vi "TDMS logging.vi"(8 "error in (no error)":errorcluster, 9 "Data":ext[][](array[numeric]), 10 "Default TDMS path":string, 11 "logg ON/OFF":bool) -> (0 "error out":errorcluster, 3 "Logg path":path)   [LabVIEW 2014]
uses:
  Ctrls/TDMS logg state.ctl
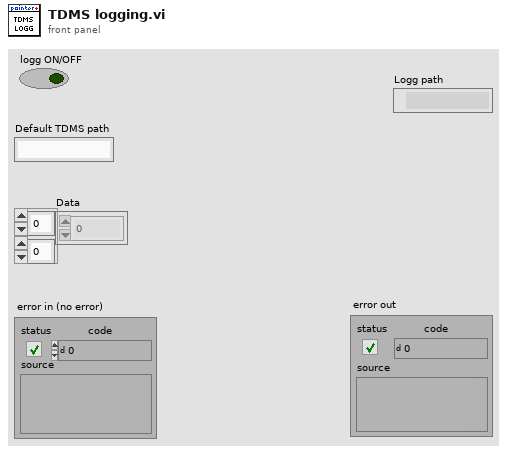
[diagram p1: front panel]
types:
  T1 = typedef "TDMS logg state.ctl" = enum16{"start", "logg", "end", "none"}
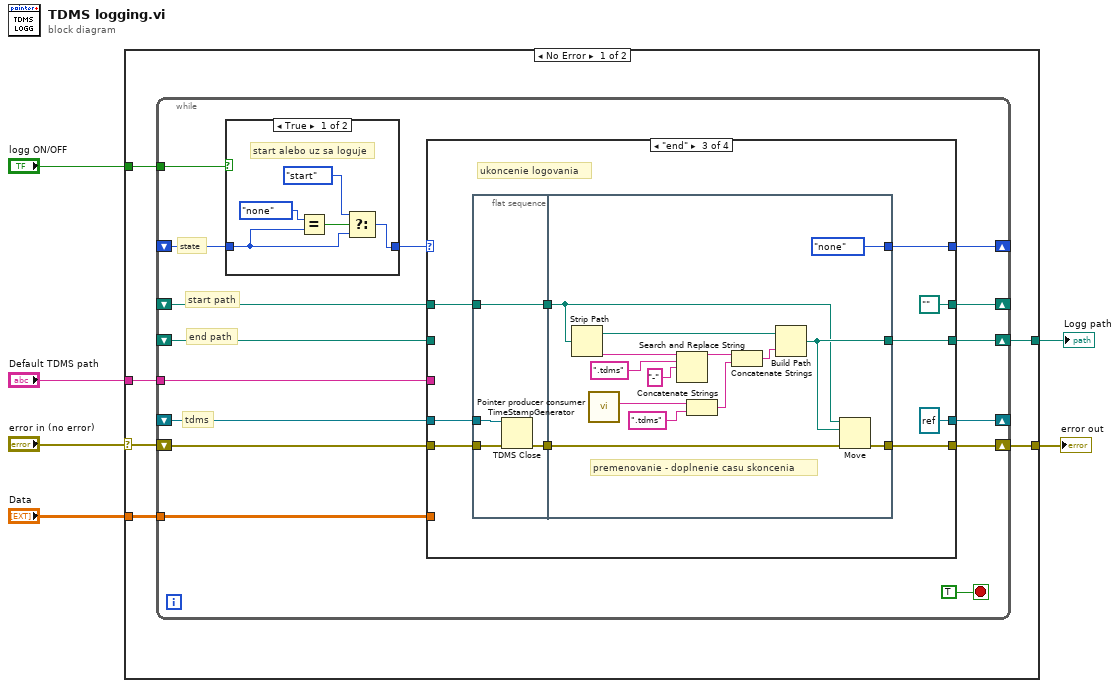
[diagram p0: block diagram]
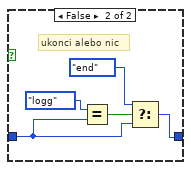
[diagram p2: hidden frame]
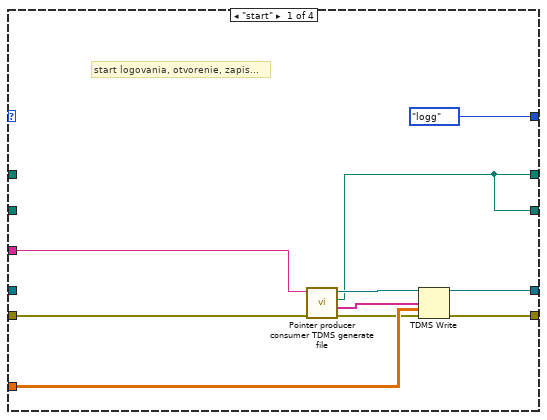
[diagram p3: hidden frame]
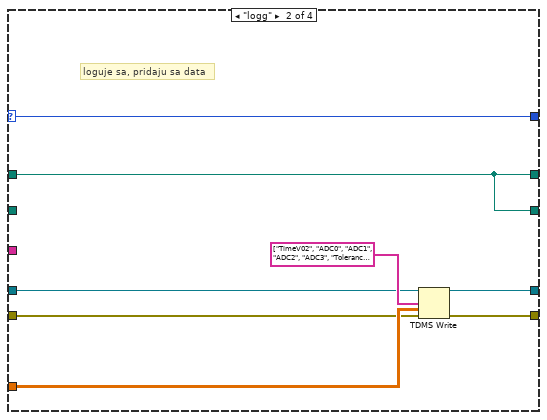
[diagram p4: hidden frame]
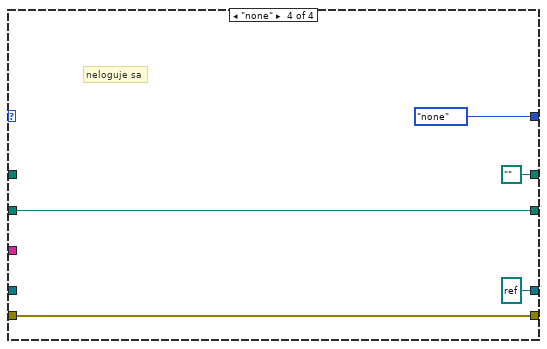
[diagram p5: hidden frame]
diagram:
  n1 = case shown="No Error" "error in (no error)" {
    selector: "error in (no error)" -> [w7 w89]
    tunnel: [w12 _] -> w6
    tunnel: "Default TDMS path" -> [w11 _]
    tunnel: "logg ON/OFF" -> [w10 _]
    tunnel: "Data" -> [w9 _]
    tunnel: [w8 w89] -> w2
    frame No Error {
      n2 = while {
        tunnel: w11 -> [w26]
        tunnel: w10 -> [w15]
        tunnel: w9 -> [w25]
        shift-right: [w23] -> _
        shift-left: _ -> [w22]
        shift-right: [w20] -> _
        shift-left: _ -> [w13]
        shift-right: [w21] -> w8
        shift-left: w7 -> [w19]
        shift-right: [w18] -> _
        shift-left: _ -> [w17]
        shift-right: [w27] -> w12
        shift-left: _ -> [w16]
        stop <- TRUE stop-if-true
        # "end path"
        # "start path"
        # "state"
        # "tdms"
        n3 = case shown="True" w15 {
          tunnel: [w29 w34] -> w14
          tunnel: w13 -> [w30 w35]
          frame True {
            # "start alebo uz sa loguje"
            n4 = Equal?(x=TDMS_logg_state."none", y=w30) -> (x = y?=w31:bool)
            n5 = Select(t=TDMS_logg_state."start", s=w31, f=w30) -> (s? t:f=w29:T1)
          }
          frame False {
            # "ukonci alebo nic"
            n6 = Equal?(x=TDMS_logg_state."logg", y=w35) -> (x = y?=w36:bool)
            n7 = Select(t=TDMS_logg_state."end", s=w36, f=w35) -> (s? t:f=w34:T1)
          }
        }
        n8 = case shown="\"end\"" w14 {
          selector: w14 -> [_ w48 _ _]
          tunnel: w25 -> [w46 w55 _ _]
          tunnel: w26 -> [w47 _ _ _]
          tunnel: [w44 w53 refnum<k34> refnum ("tdms file out") refnum<k34> refnum ("tdms file out")] -> w23
          tunnel: [w39 w49 w65 w85] -> w27
          tunnel: w22 -> [_ w52 w62 _]
          tunnel: [w41 w51 w63 w88] -> w21
          tunnel: [TDMS_logg_state."logg" w48 w61 TDMS_logg_state."none"] -> w20
          tunnel: w19 -> [w38 w50 w64 w88]
          tunnel: [w39 w49 path "" ("path") path "" ("path")] -> w18
          tunnel: w17 -> [_ w49 w60 _]
          tunnel: w16 -> [_ _ _ w85]
          frame "start" {
            # "start logovania, otvorenie, zapis..."
            n9 = call "Pointer producer consumer TDMS generate file.vi"("error in (no error)"=w38, "Default Folder Path"=w47) -> ("error out"=w43:errorcluster, "channel name(s)"=w45:string[], "path"=w39:path, "tdms file out"=w42:refnum<k34>)  [unwired: 5 in]
            n10 = TDMS Write(0:w42, 7:w45, 9:w46, 11:w43) -> (4:w44:refnum<k34>, 15:w41:errorcluster)  [unwired: 2 in, 2 out]
          }
          frame "logg" {
            # "loguje sa, pridaju sa data"
            n11 = TDMS Write(0:w52, 7:string[] ["TimeV02", "ADC0", "ADC1", "ADC2", "ADC3", "Tolerance", "CD_User", "CD_Act", "CD_Value", "Loopback", "Down", "Up", "Right", "Left", "Moving", "Loops"] ("channel name(s) in (Untitled)"), 9:w55, 11:w50) -> (4:w53:refnum<k34>, 15:w51:errorcluster)  [unwired: 2 in, 2 out]
          }
          frame "end" {
            # "ukoncenie logovania"
            n12 = flat-sequence {
              tunnel: w64 -> [w69]
              tunnel: [w68] -> w57
              tunnel: w62 -> [w67]
              tunnel: w60 -> [w66]
              tunnel: [w66] -> w56
              tunnel: [w74] -> w65
              tunnel: [w72] -> w63
              tunnel: w57 -> [w73]
              tunnel: [TDMS_logg_state."none"] -> w61
              tunnel: w56 -> [w70]
              frame #0 {
                n13 = TDMS Close(8:w69, 11:w67) -> (0:w68:errorcluster)  [unwired: 1 out]
              }
              frame #1 {
                # "premenovanie - doplnenie casu skoncenia"
                n14 = Strip Path(path=w70) -> (stripped path=w81:path, name=w80:string)
                n15 = call "Pointer producer consumer TimeStampGenerator.vi"() -> ("Local time (HHMMSS)"=w82:string)  [unwired: 8 in, 2 out]
                n16 = Search and Replace String(input string=w80, search string=".tdms", replace string="-" ("replace string (\"\")")) -> (result string=w77:string)  [unwired: 5 in, 3 out]
                n17 = Concatenate Strings(w82, ".tdms") -> (w76:string)
                n18 = Concatenate Strings(w77, w76) -> (w75:string)
                n19 = Build Path(base path=w81, name or relative path=w75) -> (appended path=w74:path)
                n20 = Move(source path=w70, error in=w73, 10:w74) -> (error out=w72:errorcluster)  [unwired: 2 in, 2 out]
              }
            }
          }
          frame "none" {
            # "neloguje sa"
          }
        }
      }
    }
    frame Error {
    }
  }
  "Logg path" <- w6
  "error out" <- w2
